vi "Create PWM Output Module.vi"(8 "error in (no error)":errorcluster, 10 "channel settings":T1[](array[typedef]), 11 "module in":refnum<class "Module.lvclass">) -> (0 "error out":errorcluster, 3 "module out":refnum<class "Module.lvclass">)   [LabVIEW 2017, in "Scan Engine Scripting.lvlib" / "Module.lvclass"]
uses:
  Module.lvclass
  Mode Classes/Controls/pwm channel settings.ctl
  Channel Classes/PWM Output Channel/Frequency.ctl
  Mode Classes/PWM Mode/PWM Mode.lvclass
  C:/Users/nitest/Documents/niveristand-scan-engine-ethercat-custom-device/Custom Device Source/Scripting/Modules/Mode Classes/Mode/Mode.lvclass
  Channel Classes/PWM Output Channel/PWM Output Channel.lvclass
  C:/Users/nitest/Documents/niveristand-scan-engine-ethercat-custom-device/Custom Device Source/Scripting/Modules/Channel Classes/Channel/Channel.lvclass
  Scan Engine Scripting.lvlib
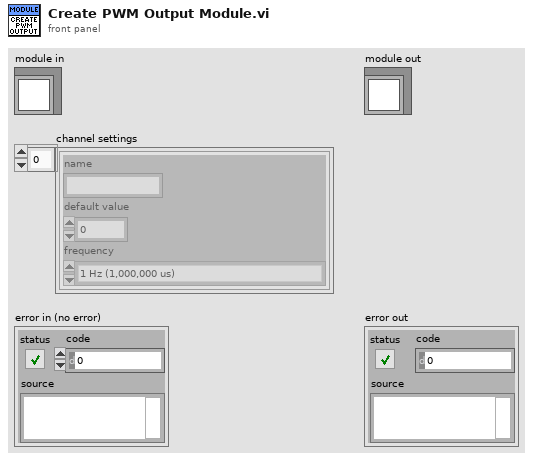
[diagram p1: front panel]
types:
  T1 = typedef "Scan Engine Scripting.lvlib/pwm channel settings.ctl" = cluster{"name":string, "default value":dbl, "frequency":T2}
  T2 = typedef "Scan Engine Scripting.lvlib/PWM Output Channel.lvclass/Frequency.ctl" = enum16{"1 Hz (1,000,000 us)", "50 Hz (20,000 us)", "250 Hz (4,000 us)", "500 Hz (2,000 us)", "1 kHz (1,000 us)", "5 kHz (200 us)", "10 kHz (100 us)", "20 kHz (50 us)"}
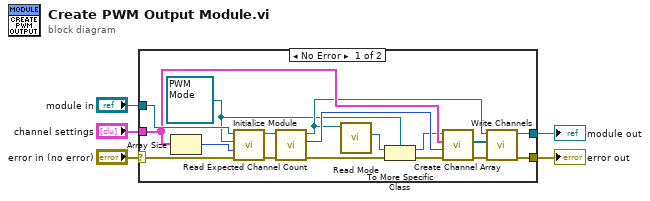
[diagram p0: block diagram]
diagram:
  n1 = case shown="No Error" "error in (no error)" {
    selector: "error in (no error)" -> [w22 w24]
    tunnel: [w19 w24] -> w2
    tunnel: [w20 w23] -> w4
    tunnel: "module in" -> [w21 w23]
    tunnel: "channel settings" -> [w13 _]
    frame No Error {
      w9 = refnum<class "PWM Mode.lvclass"> refnum ("Scan Engine Scripting.lvlib:PWM Mode.lvclass")
      n2 = Array Size(array=w13) -> (size(s)=w12:i32)
      n3 = call-dynamic "Initialize Module.vi"("error in"=w22, "channel array size"=w12, "mode"=w9, "module in"=w21) -> ("error out"=w17:errorcluster, "module out"=w18:refnum<class "Module.lvclass">)  [unwired: 6 in]
      n4 = call-dynamic "Read Expected Channel Count.vi"("error in"=w17, "module in"=w18) -> ("error out"=w7:errorcluster, "expected channel count"=w14:i32, "module out"=w11:refnum<class "Module.lvclass">)  [unwired: 7 in]
      n5 = call-dynamic "Read Mode.vi"("module in"=w11) -> ("mode"=w10:refnum<class "Mode.lvclass">)  [unwired: 8 in, 2 out]
      n6 = To More Specific Class(target class=w9, reference=w10, error in=w7) -> (specific class reference=w8:refnum<class "PWM Mode.lvclass">, error out=w6:errorcluster)
      n7 = call "Create Channel Array.vi"("error in"=w6, "expected channel count"=w14, "channel settings"=w13, "PWM Mode in"=w8) -> ("error out"=w16:errorcluster, "channels"=w15:refnum<class "PWM Output Channel.lvclass">[])  [unwired: 5 in, 1 out]
      n8 = call-dynamic "Write Channels.vi"("error in"=w16, "channels"=w15, "module in"=w11) -> ("error out"=w19:errorcluster, "module out"=w20:refnum<class "Module.lvclass">)  [unwired: 7 in]
    }
    frame Error {
    }
  }
  "module out" <- w4
  "error out" <- w2
